vi "暂停or运行.vi"() -> ()   [LabVIEW 2011]
panel:
  out "Numeric":i32
  out "Waveform Chart":dbl(graph)
  in  "暂停":bool
  in  "stop":bool
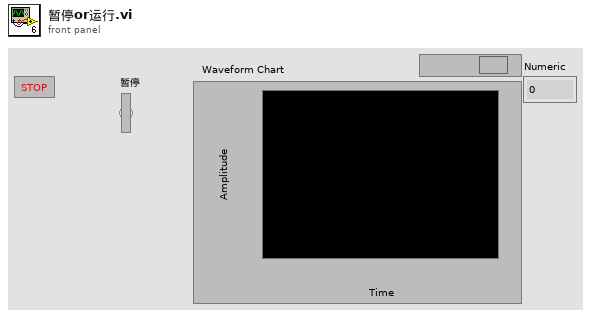
[diagram p1: front panel]
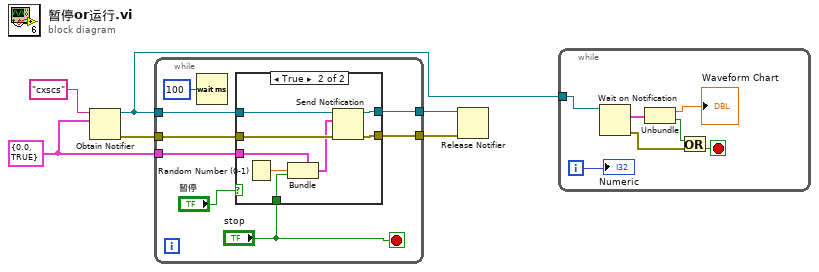
[diagram p0: block diagram]
diagram:
  w2 = cluster{dbl, bool} {0.0, TRUE}
  n1 = Obtain Notifier(name (unnamed)="cxscs", notification data type=w2) -> (notifier out=w1:refnum<notifier>, error out=w5:errorcluster)  [unwired: 2 in, 1 out]
  n2 = while {
    tunnel: w1 -> [w14]
    tunnel: w5 -> [w13]
    tunnel: [w12] -> w4
    tunnel: [w11] -> w3
    tunnel: w2 -> [w9]
    stop <- "stop" stop-if-true
    n3 = Wait (ms)(milliseconds to wait=u32 100) -> ()  [unwired: 1 out]
    n4 = case shown="True" "暂停" {
      tunnel: w14 -> [w16 w24]
      tunnel: w13 -> [w15 w23]
      tunnel: [w16 w22] -> w12
      tunnel: [w15 w21] -> w11
      tunnel: w9 -> [_ w20]
      tunnel: "stop" -> [_ w17]
      frame False {
      }
      frame True {
        n5 = Random Number (0-1)() -> (number: 0 to 1=w19:dbl)
        n6 = Bundle(cluster=w20, w19, w17) -> (w18:cluster{dbl, bool})
        n7 = Send Notification(notification=w18, notifier=w24, error in (no error)=w23) -> (notifier out=w22:refnum<notifier>, error out=w21:errorcluster)
      }
    }
  }
  n8 = Release Notifier(notifier=w4, error in (no error)=w3) -> ()  [unwired: 1 in, 3 out]
  n9 = while {
    tunnel: w1 -> [w31]
    i -> [w25]
    stop <- w28 stop-if-true
    n10 = Wait on Notification(notifier=w31) -> (notification=w30:cluster{dbl, bool}, error out=w26:errorcluster)  [unwired: 3 in, 2 out]
    n11 = Unbundle(w30) -> (→"Waveform Chart":dbl, w27:bool)
    n12 = Or(x=w27, y=w26) -> (x .or. y?=w28:bool)
    "Numeric" <- w25
  }
